vi "Write Root Parallel Operation Period(ms).vi"(8 "error in (no error)":errorcluster, 10 "Root Parallel Operation Period(ms)":i32=100, 11 "Parallel Operation Root Actor in":refnum<class "Parallel Operation Root Actor.lvclass">) -> (0 "error out":errorcluster, 3 "Parallel Operation Root Actor out":refnum<class "Parallel Operation Root Actor.lvclass">)   [LabVIEW 2024, in "Parallel Operation Root Actor.lvclass"]
uses:
  Parallel Operation Root Actor.lvclass
  Parallel Operation Root Actor.lvclass/Parallel Operation Root Actor.ctl
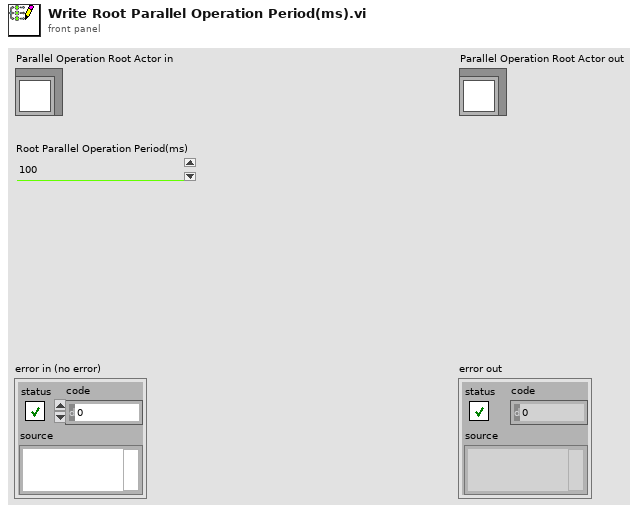
[diagram p1: front panel]
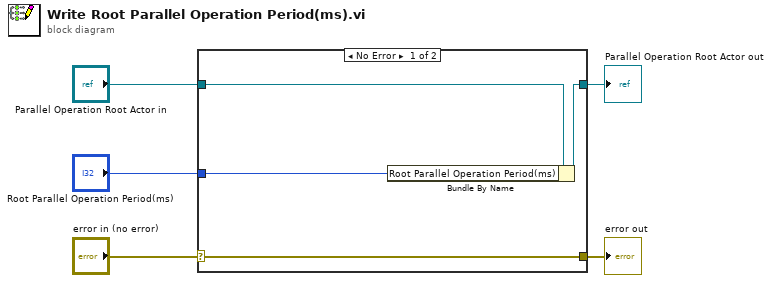
[diagram p0: block diagram]
diagram:
  n1 = case shown="No Error" "error in (no error)" {
    selector: "error in (no error)" -> [w9 w10]
    tunnel: [w9 w10] -> w4
    tunnel: [w7 w11] -> w2
    tunnel: "Parallel Operation Root Actor in" -> [w8 w11]
    tunnel: "Root Parallel Operation Period(ms)" -> [w6 _]
    frame No Error {
      n2 = Bundle By Name(cluster=w8, "Root Parallel Operation Period(ms)"=w6) -> (w7:refnum<class "Parallel Operation Root Actor.lvclass">)
    }
    frame Error {
    }
  }
  "error out" <- w4
  "Parallel Operation Root Actor out" <- w2
